vi "TMP007 Init.vi"(7 "I2C Channel":u8=1, 8 "error in (no error)":errorcluster, 9 "Samples to Average":u16(ring) items=["1 sample, .26s conversion"=0, "2 samples, .51s conversion"=512, "4 samples, 1.01s conversion"=1024, "8 samples, 2.01s conversion"=1536, "16 samples, 4.01s conversion"=2048], 10 "I2C Slave Address":u8=119 format="%.0x", 11 "LINX Resource in":T1) -> (0 "error out":errorcluster, 3 "LINX Resource out":T1)   [LabVIEW 2014]
uses:
  <vilib>/MakerHub/LINX/Private/Type Defs/LINX Ref.ctl
  <vilib>/MakerHub/LINX/Private/Type Defs/Platform.ctl
  <vilib>/MakerHub/LINX/Private/Type Defs/Interface.ctl
  <vilib>/MakerHub/LINX/Private/Device/Type Defs/LINX Device Config.ctl
  <vilib>/MakerHub/LINX/Private/Device/Type Defs/TCP Config.ctl
  <vilib>/MakerHub/LINX/Private/Device/Type Defs/Channels.ctl
  <vilib>/MakerHub/LINX/Private/Local IO/LinxI2cWrite.vi
  <vilib>/MakerHub/LINX/Public/Utilities/Check Channel.vi
  <vilib>/myRIO/Instrument Drivers/Onboard IO/I2C/vis/Write.vi
  <vilib>/MakerHub/LINX/Private/Utilties/Generate Error.vi
  <vilib>/MakerHub/LINX/Private/Utilties/Channel FGVs/I2C Channels.vi
  <vilib>/Utility/error.llb/Error Cluster From Error Code.vi
  <vilib>/myRIO/Common/Instrument Driver Framework/myRIO v1.0/I2C/vis/myRIO v1.0 Write I2C.vi
  <vilib>/MakerHub/LINX/LMH-LINX.lvlib
  <vilib>/MakerHub/LINX/Private/Device/Device.lvlib
panel:
  # "Each sample takes .25s to convert\nThere are some other conversion modes that include idle times, but I didn't include those modes"
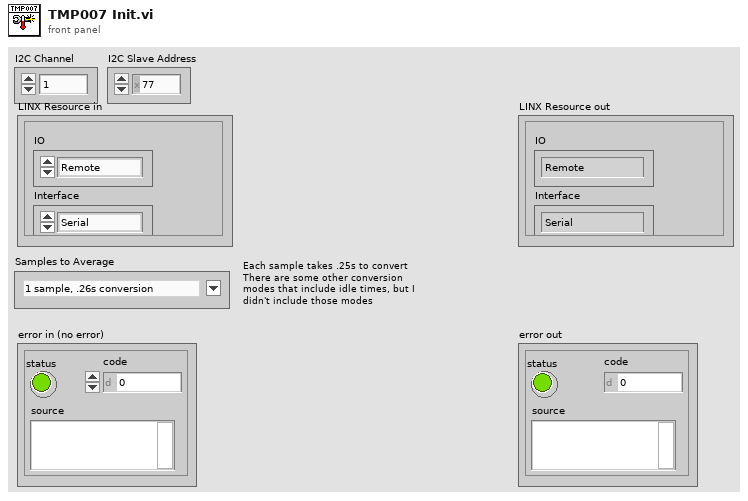
[diagram p1: front panel]
types:
  T1 = typedef "LMH-LINX.lvlib/LINX Ref.ctl" = cluster{"IO":T2, "Interface":T3, "LINX Device Config":T4}
  T2 = typedef "LMH-LINX.lvlib/Platform.ctl" = enum16{"Remote", "Local"}
  T3 = typedef "LMH-LINX.lvlib/Interface.ctl" = enum16{"Serial", "TCP"}
  T4 = typedef "LMH-LINX.lvlib/Device.lvlib/LINX Device Config.ctl" = cluster{"Interface":T3, "COM Port":refnum<visa-resource-name>, "TCP Configuration":T5, "Device Family":u8, "Device ID":u8, "Device Name":string, "TCP Ref":refnum<k5>, "Channels":T6}
  T5 = typedef "LMH-LINX.lvlib/Device.lvlib/TCP Config.ctl" = cluster{"IP Address":string, "Port":u16}
  T6 = typedef "LMH-LINX.lvlib/Channels.ctl" = cluster{"DI":u8[], "DO":u8[], "AI":u8[], "AO":u8[], "PWM":u8[], "QE":u8[], "UART":u8[], "I2C 2":u8[], "SPI":u8[], "CAN":u8[], "Servo":u8[], "AI Ref (V)":dbl, "AI Resolution (Bits)":u8, "AO Ref (V)":dbl, "AO Resolution (Bits)":u8}
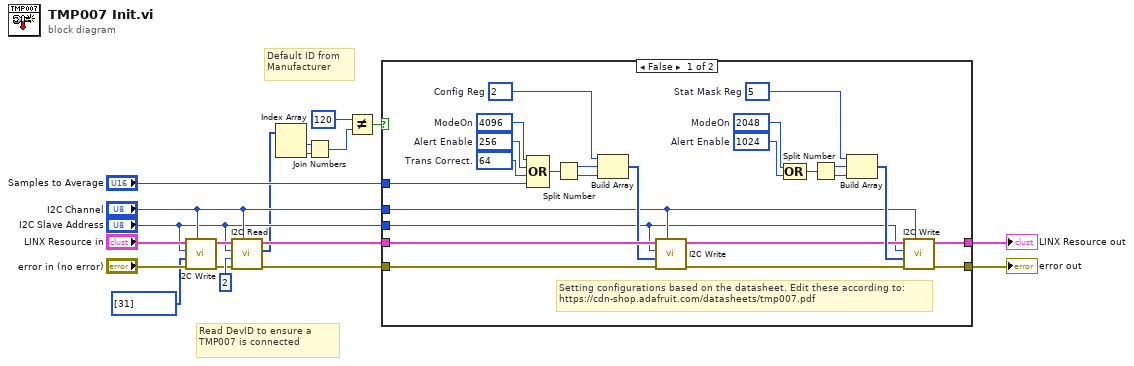
[diagram p0: block diagram]
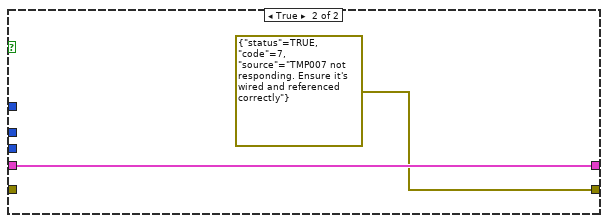
[diagram p2: hidden frame]
diagram:
  # "Default ID from Manufacturer"
  # "Read DevID to ensure a TMP007 is connected"
  n1 = call <vilib>:"I2C Write.vi"("I2C Channel"="I2C Channel", "Error In"="error in (no error)", "Data"=u8[] [31], "I2C Slave Address (0)"="I2C Slave Address", "LINX Resource"="LINX Resource in") -> ("Error Out"=w12:errorcluster, "LINX Resource"=w11:T1)  [unwired: 5 in]
  n2 = call <vilib>:"I2C Read.vi"("I2C Channel"="I2C Channel", "Error In"=w12, "Bytes To Read"=u8 2, "I2C Slave Address (0)"="I2C Slave Address", "LINX Resource"=w11) -> ("Error Out"=w15:errorcluster, "Data"=w5:u8[], "LINX Resource"=w16:T1)  [unwired: 4 in]
  n3 = Index Array(array=w5) -> (element #1=w3:u8, element #2=w4:u8)  [unwired: 2 in]
  n4 = Join Numbers(hi=w3, lo=w4) -> ((hi.lo)=w2:u16)
  n5 = Not Equal?(x=u16 120, y=w2) -> (x != y?=w9:bool)
  n6 = case shown="False" w9 {
    tunnel: w16 -> [w43 w45]
    tunnel: [w21 w45] -> w18
    tunnel: w15 -> [w42 _]
    tunnel: [w20 errorcluster {"status"=TRUE, "code"=7, "source"="TMP007 not responding. Ensure it's wired and referenced correctly"} ("error constant")] -> w17
    tunnel: "Samples to Average" -> [w41 _]
    tunnel: "I2C Channel" -> [w23 _]
    tunnel: "I2C Slave Address" -> [w22 _]
    frame False {
      w32 = u8 5  # Stat Mask Reg
      w27 = u16 1024  # Alert Enable
      w28 = u16 2048  # ModeOn
      w34 = u8 2  # Config Reg
      w40 = u16 64  # Trans Correct.
      w39 = u16 256  # Alert Enable
      w38 = u16 4096  # ModeOn
      # "Setting configurations based on the datasheet. Edit these according to:\nhttps://cdn-shop.adafruit.com/datasheets/tmp007.pdf"
      n7 = Compound Arithmetic op=OR(w38, w39, w40, w41) -> (w37:u16)
      n8 = Split Number(x=w37) -> (hi(x)=w36:u8, lo(x)=w35:u8)
      n9 = Build Array(w34, w36, w35) -> (w33:u8[])
      n10 = call <vilib>:"I2C Write.vi"("I2C Channel"=w23, "Error In"=w42, "Data"=w33, "I2C Slave Address (0)"=w22, "LINX Resource"=w43) -> ("Error Out"=w24:errorcluster, "LINX Resource"=w25:T1)  [unwired: 5 in]
      n11 = Compound Arithmetic op=OR(w28, w27) -> (w29:u16)
      n12 = Split Number(x=w29) -> (hi(x)=w30:u8, lo(x)=w31:u8)
      n13 = Build Array(w32, w30, w31) -> (w26:u8[])
      n14 = call <vilib>:"I2C Write.vi"("I2C Channel"=w23, "Error In"=w24, "Data"=w26, "I2C Slave Address (0)"=w22, "LINX Resource"=w25) -> ("Error Out"=w20:errorcluster, "LINX Resource"=w21:T1)  [unwired: 5 in]
    }
    frame True {
    }
  }
  "error out" <- w17
  "LINX Resource out" <- w18
